vi "Generate Error.vi"(4 "source level (1)":i32=1, 5 "match code":i32=2147483647, 6 "status type (error:T)":bool=TRUE, 7 "error code (-1301)":i32=-1301, 8 "error in":errorcluster, 10 "description":string) -> (0 "error out":errorcluster)   [LabVIEW 2018, in "STEPkgDriver_LINC.lvlib"]
doc: "Generates a user-defined error in the \"error out\" cluster."
uses:
  STEPkgDriver_LINC.lvlib
panel:
  # "error\nwarning"
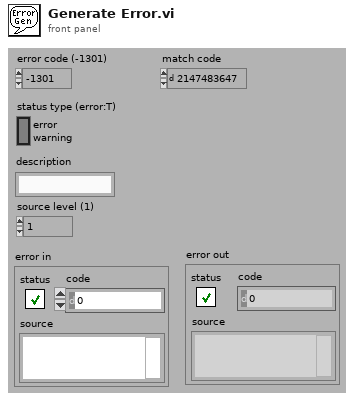
[diagram p1: front panel]
types:
  T1 = cluster{"status type (error:T)":bool, "error code (-1301)":i32, string}
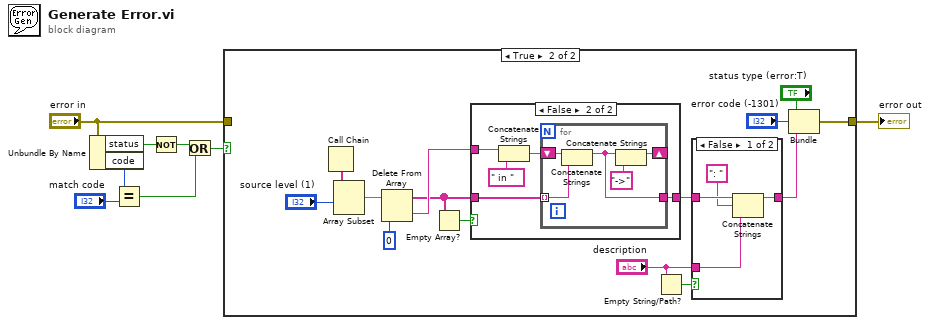
[diagram p0: block diagram]
diagram:
  n1 = Unbundle By Name("error in") -> ("status"=w6:bool, "code"=w8:i32)
  n2 = Equal?(x=w8, y="match code") -> (x = y?=w4:bool)
  n3 = Not(x=w6) -> (.not. x?=w5:bool)
  n4 = Or(x=w5, y=w4) -> (x .or. y?=w3:bool)
  n5 = case shown="True" w3 {
    tunnel: [w9 w23] -> w1
    tunnel: "error in" -> [w9 _]
    frame False {
    }
    frame True {
      n6 = Call Chain() -> (call chain=w19:string[])
      n7 = Array Subset(array=w19, index="source level (1)") -> (w14:string[])  [unwired: 1 in]
      n8 = Delete From Array(array=w14, index=0) -> (deleted portion=w12:string, array with subset deleted=w11:string[])  [unwired: 1 in]
      n9 = Empty Array?(array=w11) -> (empty?=w10:bool)
      n10 = case shown="False" w10 {
        tunnel: [w29 w34] -> w18
        tunnel: w11 -> [_ w33]
        tunnel: w12 -> [w29 w32]
        frame True {
        }
        frame False {
          n11 = Concatenate Strings(w32, " in ") -> (w30:string)
          n12 = for {
            shift-right: [w37] -> _
            shift-left: w30 -> [w39]
            tunnel: w33 -> [w38] mode=indexing
            tunnel: [w35] -> w34
            n13 = Concatenate Strings(w39, w38) -> (w35:string)
            n14 = Concatenate Strings(w35, "->") -> (w37:string)
          }
        }
      }
      n15 = Empty String/Path?(string/path="description") -> (empty?=w17:bool)
      n16 = case shown="False" w17 {
        tunnel: w18 -> [w27 w28]
        tunnel: "description" -> [w26 _]
        tunnel: [w24 w28] -> w15
        frame False {
          n17 = Concatenate Strings(w27, ": ", w26) -> (w24:string)
        }
        frame True {
        }
      }
      n18 = Bundle("status type (error:T)"="status type (error:T)", "error code (-1301)"="error code (-1301)", w15) -> (w23:T1)  [unwired: 1 in]
    }
  }
  "error out" <- w1
